vi "HEWH Get UEF.vi"(6 "Maufacturing Date":T1(ring), 7 "Water Heater Type":T7, 8 "error in (no error)":errorcluster, 10 "UEF Calculated Values":T2 {"Data Indexes"."15 sec after Draw Index" format="%#.2f"; "Data Indexes"."15 sec after Draw Timestamp" format="%#.2f"; "Data Indexes"."Test Start Timestamp" format="%.2f"; "Data Indexes"."Test End Timestamp" format="%.2f"; "Data Indexes"."T0 Timestamp" format="%.2f"; "Data Indexes"."Tsf Timestamp" format="%.2f"; "Data Indexes"."Tsu0 Timestamp" format="%.2f"; "Data Indexes"."Tmax1 Timestamp" format="%.2f"; "Data Indexes"."Draw Index Timestamp" format="%#.2f"; "Data Indexes"."Non-Draw Timestamp" format="%#.2f"; "Data Indexes"."Heating Timestamp" format="%#.2f"; "Data Indexes"."Start Energy (BTU-Gas)" format="%.6f"; "Data Indexes"."Start Watt Hours" format="%.6f"; "Static Data"."V - Volume of Wh (True)" format="%.5f"; "Static Data"."T-Ambinet Nominal (°F)" format="%.5f"; "Static Data"."T-Inlet Setpoint (°F)" format="%.5f"; "Static Data"."T-Wh Setpoint (°F)" format="%.5f"; "Sampled Data"."Qe (Wh)" format="%.5f"; "Sampled Data"."Tau stby2 (hr)" format="%.5f"; "Sampled Data"."Tastby2 (°F)" format="%.5f"; "Sampled Data"."Qf (BTU)" format="%.5f"; "Sampled Data"."Qe (BTU)" format="%.5f"; "Sampled Data"."Tmax1 (°F)" format="%.5f"; "Sampled Data"."T0 (°F)" format="%.5f"; "Sampled Data"."Qr (BTU)" format="%.5f"; "Sampled Data"."T 24(°F)" format="%.5f"; "Sampled Data"."T astby(°F)" format="%.5f"; "Sampled Data"."T tstby(°F)" format="%.5f"; "Sampled Data"."T su0(°F)" format="%.5f"; "Sampled Data"."T suf(°F)" format="%.5f"; "Sampled Data"."Tau stby_1 (hr)" format="%.5f"; "Sampled Data"."Qsuf (BTU)" format="%.5f"; "Sampled Data"."Qsu0 (BTU)" format="%.5f"; "Calculated Values"."Draw Bonus Volume (gal)" format="%.6f"; "Calculated Values"."Adjustment Factor" format="%.6f"; "Calculated Values"."T*avg_del(n-1)" format="%.6f"; "Calculated Values"."T*min(n-1)" format="%.6f"; "Calculated Values"."T*avg_del(n)" format="%.6f"; "Calculated Values"."Vn" format="%.6f"; "Calculated Values"."Qdm (BTU)" format="%.6f"; "Calculated Values"."QHWD (BTU)" format="%.6f"; "Calculated Values"."QHW (BTU)" format="%.6f"; "Calculated Values"."UEF" format="%.6f"; "Calculated Values"."QHW67 (BTU)" format="%.6f"; "Calculated Values"."Qda (BTU)" format="%.6f"; "Calculated Values"."Qd (BTU)" format="%.6f"; "Calculated Values"."Q (BTU)" format="%.6f"; "Calculated Values"."UA (BTU/(hr*F))" format="%.6f"; "Calculated Values"."Qhr (BTU/hr)" format="%.6f"; "Calculated Values"."Qstby (BTU)" format="%.6f"; "Calculated Values"."nu_r" format="%.6f"; "Calculated Values"."CpUEF (BTU/(lb*F))" format="%.6f"; "Calculated Values"."rho_nu (lb/gal)" format="%.6f"; "Calculated Values"."V1- Vol (Gal)" format="%.6f"; "Calculated Values"."M cluster mass removed (lb)" format="%.6f"; "Calculated Values"."Cp theoretical (BTU/(lbm °F))" format="%.6f"; "Calculated Values"."Tin1 - Mean Inlet 1st Cluster (°F)" format="%.6f"; "Calculated Values"."Tdel1-Mean Outlet 1st Cluster(°F)" format="%.6f"; "Calculated Values"."Cp 24 (BTU/(lb*F))" format="%.6f"; "Calculated Values"."Cp standby (BTU/(lb*F))" format="%.6f"; "Calculated Values"."Cp2 (BTU/(lb*F))" format="%.6f"; "Calculated Values"."Cp1 (BTU/(lb*F))" format="%.6f"; "Calculated Values"."rho 24 (lb/gal)" format="%.6f"; "Calculated Values"."rho standby (lb/gal)" format="%.6f"; "Calculated Values"."rho 2 (lb/gal)" format="%.6f"; "Calculated Values"."Density of cold water All (lbm/gal)" format="%#.3g"; "Calculated Values"."CpHW (BTU/(lbm °F))" format="%#.3g"; "Calculated Values"."Density of hot water All (lbm/gal)" format="%#.3g"; "Calculated Values"."Mass of water All (lbm)" format="%#.3f"}, 11 "24 Hour UEF Location":path) -> (0 "error out":errorcluster, 2 "UEF Calculated Values Output":T2 {"Data Indexes"."15 sec after Draw Index" format="%#.2f"; "Data Indexes"."15 sec after Draw Timestamp" format="%#.2f"; "Data Indexes"."Test Start Timestamp" format="%.2f"; "Data Indexes"."Test End Timestamp" format="%.2f"; "Data Indexes"."T0 Timestamp" format="%.2f"; "Data Indexes"."Tsf Timestamp" format="%.2f"; "Data Indexes"."Tsu0 Timestamp" format="%.2f"; "Data Indexes"."Tmax1 Timestamp" format="%.2f"; "Data Indexes"."Draw Index Timestamp" format="%#.2f"; "Data Indexes"."Non-Draw Timestamp" format="%#.2f"; "Data Indexes"."Heating Timestamp" format="%#.2f"; "Data Indexes"."Start Energy (BTU-Gas)" format="%.6f"; "Data Indexes"."Start Watt Hours" format="%.6f"; "Static Data"."V - Volume of Wh (True)" format="%.5f"; "Static Data"."T-Ambinet Nominal (°F)" format="%.5f"; "Static Data"."T-Inlet Setpoint (°F)" format="%.5f"; "Static Data"."T-Wh Setpoint (°F)" format="%.5f"; "Sampled Data"."Qe (Wh)" format="%.5f"; "Sampled Data"."Tau stby2 (hr)" format="%.5f"; "Sampled Data"."Tastby2 (°F)" format="%.5f"; "Sampled Data"."Qf (BTU)" format="%.5f"; "Sampled Data"."Qe (BTU)" format="%.5f"; "Sampled Data"."Tmax1 (°F)" format="%.5f"; "Sampled Data"."T0 (°F)" format="%.5f"; "Sampled Data"."Qr (BTU)" format="%.5f"; "Sampled Data"."T 24(°F)" format="%.5f"; "Sampled Data"."T astby(°F)" format="%.5f"; "Sampled Data"."T tstby(°F)" format="%.5f"; "Sampled Data"."T su0(°F)" format="%.5f"; "Sampled Data"."T suf(°F)" format="%.5f"; "Sampled Data"."Tau stby_1 (hr)" format="%.5f"; "Sampled Data"."Qsuf (BTU)" format="%.5f"; "Sampled Data"."Qsu0 (BTU)" format="%.5f"; "Calculated Values"."Draw Bonus Volume (gal)" format="%.6f"; "Calculated Values"."Adjustment Factor" format="%.6f"; "Calculated Values"."T*avg_del(n-1)" format="%.6f"; "Calculated Values"."T*min(n-1)" format="%.6f"; "Calculated Values"."T*avg_del(n)" format="%.6f"; "Calculated Values"."Vn" format="%.6f"; "Calculated Values"."Qdm (BTU)" format="%.6f"; "Calculated Values"."QHWD (BTU)" format="%.6f"; "Calculated Values"."QHW (BTU)" format="%.6f"; "Calculated Values"."UEF" format="%.6f"; "Calculated Values"."QHW67 (BTU)" format="%.6f"; "Calculated Values"."Qda (BTU)" format="%.6f"; "Calculated Values"."Qd (BTU)" format="%.6f"; "Calculated Values"."Q (BTU)" format="%.6f"; "Calculated Values"."UA (BTU/(hr*F))" format="%.6f"; "Calculated Values"."Qhr (BTU/hr)" format="%.6f"; "Calculated Values"."Qstby (BTU)" format="%.6f"; "Calculated Values"."nu_r" format="%.6f"; "Calculated Values"."CpUEF (BTU/(lb*F))" format="%.6f"; "Calculated Values"."rho_nu (lb/gal)" format="%.6f"; "Calculated Values"."V1- Vol (Gal)" format="%.6f"; "Calculated Values"."M cluster mass removed (lb)" format="%.6f"; "Calculated Values"."Cp theoretical (BTU/(lbm °F))" format="%.6f"; "Calculated Values"."Tin1 - Mean Inlet 1st Cluster (°F)" format="%.6f"; "Calculated Values"."Tdel1-Mean Outlet 1st Cluster(°F)" format="%.6f"; "Calculated Values"."Cp 24 (BTU/(lb*F))" format="%.6f"; "Calculated Values"."Cp standby (BTU/(lb*F))" format="%.6f"; "Calculated Values"."Cp2 (BTU/(lb*F))" format="%.6f"; "Calculated Values"."Cp1 (BTU/(lb*F))" format="%.6f"; "Calculated Values"."rho 24 (lb/gal)" format="%.6f"; "Calculated Values"."rho standby (lb/gal)" format="%.6f"; "Calculated Values"."rho 2 (lb/gal)" format="%.6f"; "Calculated Values"."Density of cold water All (lbm/gal)" format="%#.3g"; "Calculated Values"."CpHW (BTU/(lbm °F))" format="%#.3g"; "Calculated Values"."Density of hot water All (lbm/gal)" format="%#.3g"; "Calculated Values"."Mass of water All (lbm)" format="%#.3f"}, 3 "24 Hour UEF Location Output":path, 4 "Full 24 Hour UEF Data":string[][](array[string]))   [LabVIEW 2023]
uses:
  Type Definitions/HEWH Water Heater Type.ctl
  Type Definitions/UEF Constants.ctl
  Type Definitions/HEWH Draw Stats.ctl
  Type Definitions/HEWH FHR Draw Type.ctl
  Type Definitions/FHR Bins.ctl
  Type Definitions/HEWH Meter Type.ctl
  Type Definitions/HEWH Test Type.ctl
  Type Definitions/HEWH Index Type.ctl
  <vilib>/Utility/file.llb/Read Delimited Spreadsheet (string).vi
  <vilib>/Utility/file.llb/Read Delimited Spreadsheet (DBL).vi
panel:
  # "FHR"
  # "FHR"
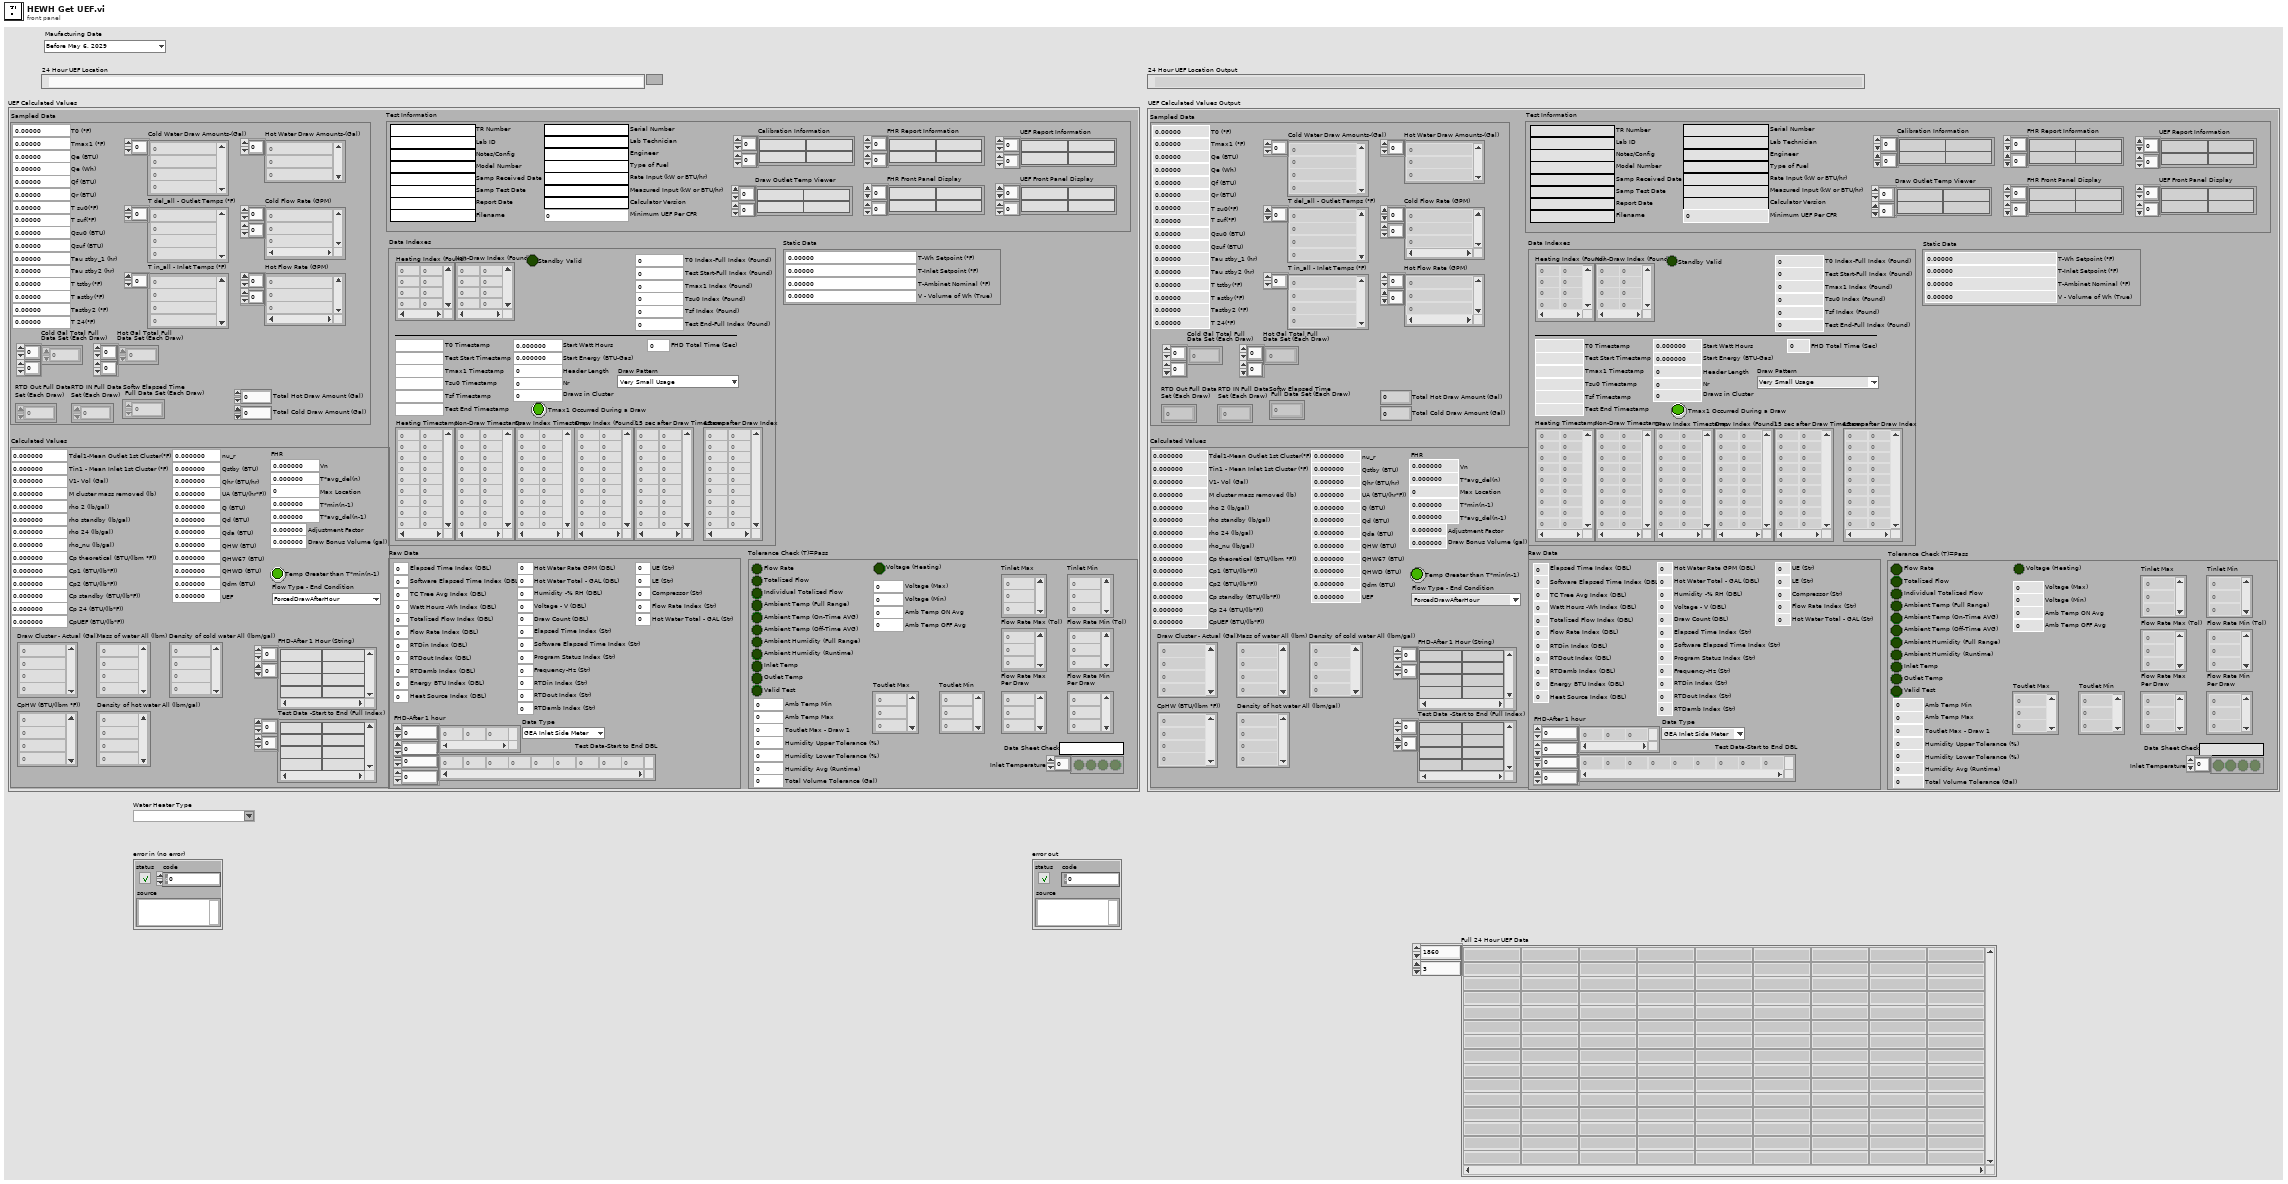
[diagram p1: front panel]
types:
  T1 = enum16{"Before May 6, 2029", "On or After May 6, 2029"}
  T2 = typedef "UEF Constants.ctl" = cluster{"Calculated Values":T3, "Sampled Data":cluster{"Cold Water Draw Amounts-(Gal)":dbl[], "T del_all - Outlet Temps (°F)":dbl[], "T in_all - Inlet Temps (°F)":dbl[], "Qsu0 (BTU)":dbl, "Qsuf (BTU)":dbl, "Tau stby_1 (hr)":dbl, "T suf(°F)":dbl, "T su0(°F)":dbl, "T tstby(°F)":dbl, "T astby(°F)":dbl, "T 24(°F)":dbl, "Qr (BTU)":dbl, "T0 (°F)":dbl, "Tmax1 (°F)":dbl, "Qe (BTU)":dbl, "Qf (BTU)":dbl, "Tastby2 (°F)":dbl, "RTD Out Full Data\nSet (Each Draw)":dbl[][], "RTD IN Full Data\nSet (Each Draw)":dbl[][], "Tau stby2 (hr)":dbl, "Hot Water Draw Amounts-(Gal)":dbl[], "Cold Flow Rate (GPM)":dbl[][], "Hot Flow Rate (GPM)":dbl[][], "Softw Elapsed Time\n Full Data Set (Each Draw)":dbl[][], "Cold Gal Total Full\nData Set (Each Draw)":dbl[][], "Total Hot Draw Amount (Gal) ":dbl, "Total Cold Draw Amount (Gal)":dbl, "Qe (Wh)":dbl, "Hot Gal Total Full\nData Set (Each Draw)":dbl[][]}, "Static Data":cluster{"T-Wh Setpoint (°F)":dbl, "T-Inlet Setpoint (°F)":dbl, "T-Ambinet Nominal (°F)":dbl, "V - Volume of Wh (True)":dbl}, "Data Indexes":cluster{"Test Start-Full Index (Found)":i32, "Header Length":i32, "Draw Index (Found)":i32[][], "Nr":i32, "Start Watt Hours":dbl, "Tsu0 Index (Found)":i32, "Tsf Index (Found)":i32, "Start Energy (BTU-Gas)":dbl, "Draws in Cluster":i32, "T0 Index-Full Index (Found)":i32, "Non-Draw Index (Found)":i32[][], "Tmax1 Index (Found)":i32, "Test End-Full Index (Found)":i32, "Heating Index (Found)":i32[][], "Heating Timestamp":dbl[][], "Non-Draw Timestamp":dbl[][], "Draw Index Timestamp":dbl[][], "Tmax1 Timestamp":dbl, "Tsu0 Timestamp":dbl, "Tsf Timestamp":dbl, "T0 Timestamp":dbl, "Test End Timestamp":dbl, "Test Start Timestamp":dbl, "15 sec after Draw Timestamp":dbl[][], "15 sec after Draw Index":dbl[][], "Tmax1 Occurred During a Draw":bool, "FHD Total Time (Sec)":dbl, "Draw Pattern":T5, "Standby Valid":bool}, "Raw Data":cluster{"Elapsed Time Index (DBL)":i32, "Software Elapsed Time Index (DBL)":i32, "TC Tree Avg Index (DBL)":i32, "Watt Hours -Wh Index (DBL)":i32, "Energy BTU Index (DBL)":i32, "Totalized Flow Index (DBL)":i32, "Flow Rate Index (DBL)":i32, "Program Status Index (Str)":i32, "RTDin Index (DBL)":i32, "RTDout Index (DBL)":i32, "RTDamb Index (DBL)":i32, "Test Data-Start to End DBL":dbl[][], "Data Type":T6, "Heat Source Index (DBL)":i32, "Hot Water Rate GPM (DBL)":i32, "Hot Water Total - GAL (DBL)":i32, "FHD-After 1 hour":dbl[][], "Humidity -% RH (DBL)":i32, "Voltage - V (DBL)":i32, "Draw Count (DBL)":i32, "Elapsed Time Index (Str)":i32, "Software Elapsed Time Index (Str)":i32, "Frequency-Hz (Str)":i32, "RTDin Index (Str)":i32, "RTDout Index (Str)":i32, "RTDamb Index (Str)":i32, "UE (Str)":i32, "LE (Str)":i32, "Compressor (Str)":i32, "Flow Rate Index (Str)":i32, "Hot Water Total - GAL (Str)":i32}, "Tolerance Check (T)=Pass":cluster{"Flow Rate":bool, "Totalized Flow":bool, "Ambient Temp (Full Range)":bool, "Ambient Humidity (Full Range)":bool, "Inlet Temp":bool, "Outlet Temp":bool, "Valid Test":bool, "Individual Totalized Flow":bool, "Data Sheet Check":string, "Inlet Temperature":bool[], "Tinlet Max":dbl[], "Tinlet Min":dbl[], "Flow Rate Max (Tol)":dbl[], "Flow Rate Min (Tol)":dbl[], "Amb Temp Max":dbl, "Amb Temp Min":dbl, "Toutlet Max - Draw 1":dbl, "Humidity Upper Tolerance (%)":dbl, "Total Volume Tolerance (Gal)":dbl, "Humidity Lower Tolerance (%)":dbl, "Flow Rate Max\nPer Draw":dbl[], "Flow Rate Min\nPer Draw":dbl[], "Ambient Humidity (Runtime)":bool, "Humidity Avg (Runtime)":dbl, "Ambient Temp (On-Time AVG)":bool, "Ambient Temp (Off-Time AVG)":bool, "Amb Temp OFF Avg":dbl, "Amb Temp ON Avg":dbl, "Voltage (Heating)":bool, "Voltage (Min)":dbl, "Voltage (Max)":dbl, "Toutlet Max":dbl[], "Toutlet Min":dbl[]}, "Test Information":cluster{"TR Number":string, "Lab ID":string, "Notes/Config":string, "Model Number":string, "Serial Number":string, "Lab Technician":string, "Engineer":string, "Type of Fuel":string, "Samp Received Date":string, "Samp Test Date":string, "Report Date":string, "Rate Input (kW or BTU/hr)":string, "Measured Input (kW or BTU/hr)":string, "Filename":string, "Calibration Information":string[][], "Calculator Version":string, "Minimum UEF Per CFR":dbl, "UEF Report Information":string[][], "FHR Report Information":string[][], "FHR Front Panel Display":string[][], "UEF Front Panel Display":string[][], "Draw Outlet Temp Viewer":string[][]}}
  T3 = typedef "HEWH Draw Stats.ctl" = cluster{"Draw Cluster - Actual (Gal)":dbl[], "Mass of water All (lbm)":dbl[], "Density of hot water All (lbm/gal)":dbl[], "CpHW (BTU/(lbm °F))":dbl[], "rho 2 (lb/gal)":dbl, "rho standby (lb/gal)":dbl, "rho 24 (lb/gal)":dbl, "Cp1 (BTU/(lb*F))":dbl, "Cp2 (BTU/(lb*F))":dbl, "Cp standby (BTU/(lb*F))":dbl, "Cp 24 (BTU/(lb*F))":dbl, "nu_r":dbl, "Qstby (BTU)":dbl, "Qhr (BTU/hr)":dbl, "UA (BTU/(hr*F))":dbl, "Q (BTU)":dbl, "Qd (BTU)":dbl, "Qda (BTU)":dbl, "QHW67 (BTU)":dbl, "UEF":dbl, "Tdel1-Mean Outlet 1st Cluster(°F)":dbl, "Tin1 - Mean Inlet 1st Cluster (°F)":dbl, "Cp theoretical (BTU/(lbm °F))":dbl, "M cluster mass removed (lb)":dbl, "V1- Vol (Gal)":dbl, "Test Data -Start to End (Full Index)":string[][], "rho_nu (lb/gal)":dbl, "Density of cold water All (lbm/gal)":dbl[], "CpUEF (BTU/(lb*F))":dbl, "QHW (BTU)":dbl, "QHWD (BTU)":dbl, "Qdm (BTU)":dbl, "FHD-After 1 Hour (String)":string[][], "Vn":dbl, "T*avg_del(n)":dbl, "Max Location":i32, "T*min(n-1)":dbl, "T*avg_del(n-1)":dbl, "Temp Greater than T*min(n-1)":bool, "Adjustment Factor":dbl, "Draw Bonus Volume (gal)":dbl, "Flow Type - End Condition":T4}
  T4 = typedef "HEWH FHR Draw Type.ctl" = enum16{"ForcedDrawAfterHour", "HeatingCutoffBeforeHour"}
  T5 = typedef "FHR Bins.ctl" = enum16{"Very Small Usage", "Low Usage", "Medium Usage", "High Usage", "Undefined"}
  T6 = typedef "HEWH Meter Type.ctl" = enum16{"GEA Inlet Side Meter", "GEA Outlet Side Meter", "CSA Inlet Side Meter"}
  T7 = typedef "HEWH Water Heater Type.ctl" = string
  T8 = typedef "HEWH Index Type.ctl" = enum16{"Draw Index", "Heating Index", "Temp Based (FHD)"}
  T9 = typedef "HEWH Test Type.ctl" = enum16{"UEF", "FHD"}
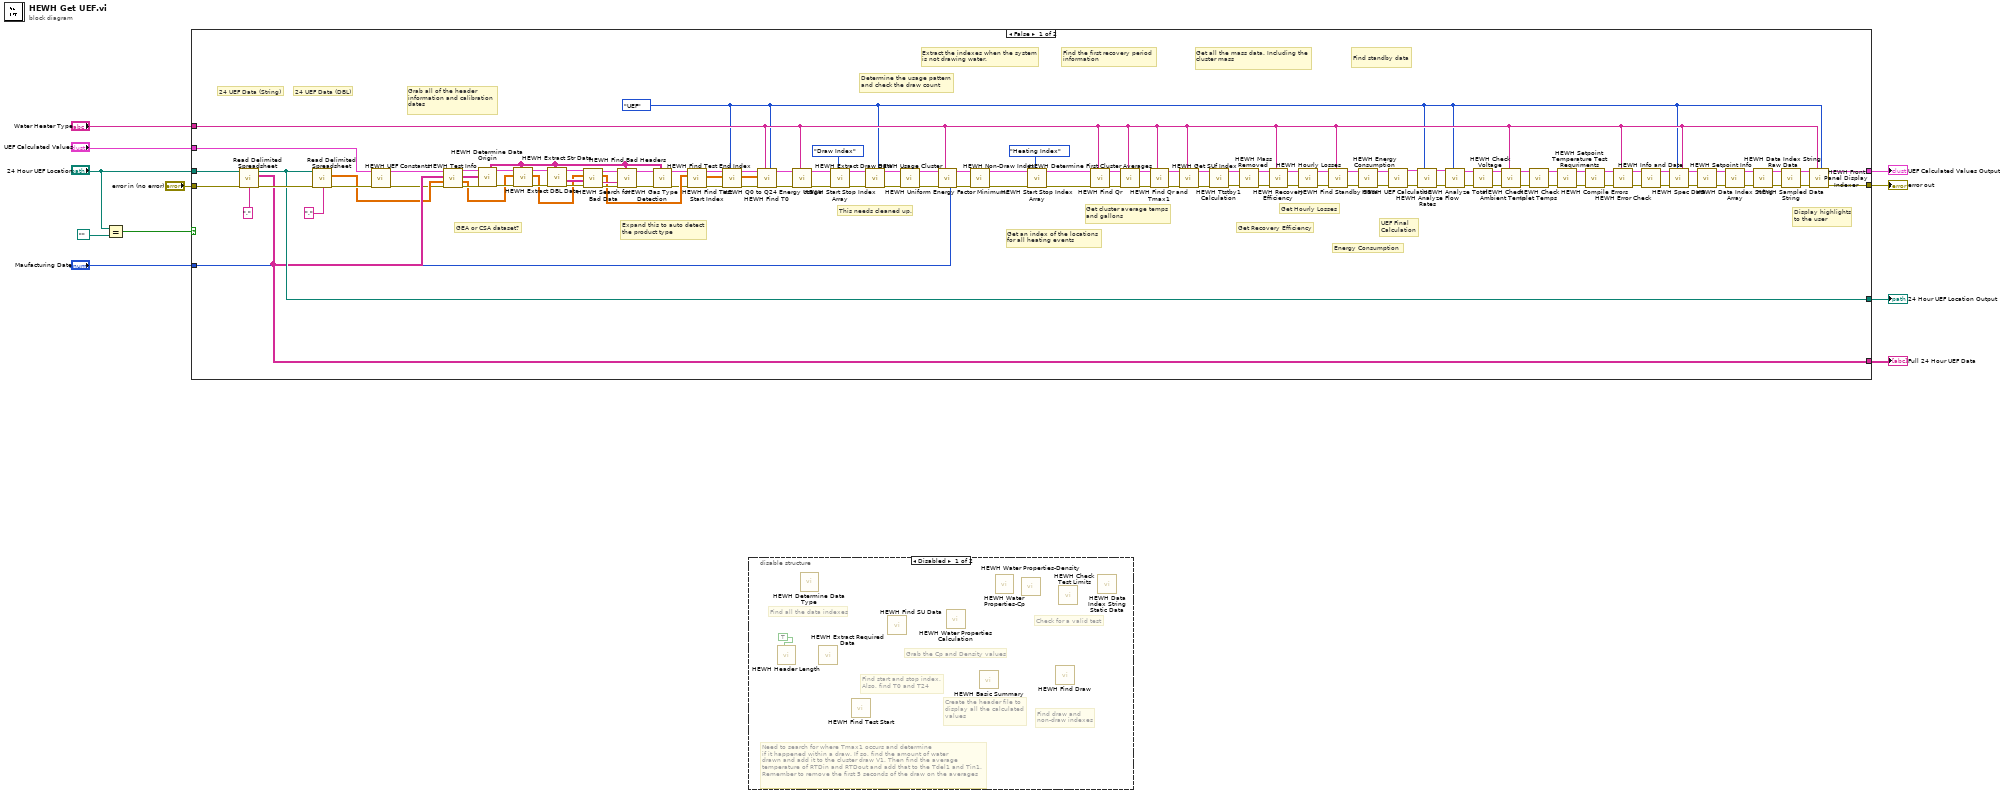
[diagram p0: block diagram]
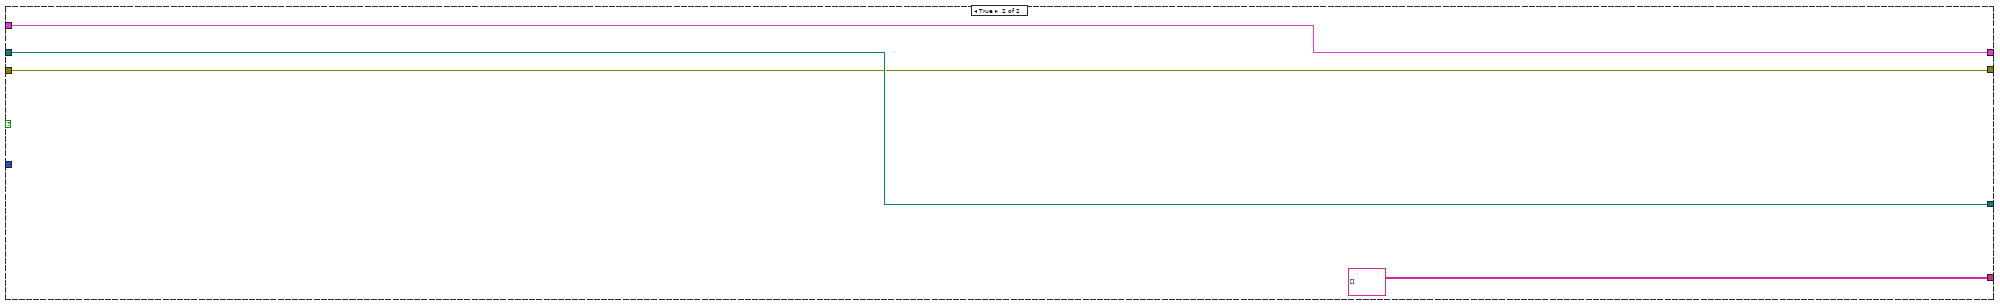
[diagram p3: hidden frame]
diagram:
  n1 = Equal?(x="24 Hour UEF Location", y=path "") -> (x = y?=w2:bool)
  n2 = case shown="False" w2 {
    tunnel: "Water Heater Type" -> [w15 _]
    tunnel: "UEF Calculated Values" -> [w88 w125]
    tunnel: [w54 string[][] [] ("all rows")] -> w9
    tunnel: "error in (no error)" -> [w123 w126]
    tunnel: [w107 w126] -> w7
    tunnel: [w12 w125] -> w6
    tunnel: [w108 w127] -> w5
    tunnel: "24 Hour UEF Location" -> [w109 w127]
    tunnel: "Maufacturing Date" -> [w46 _]
    frame False {
      w13 = HEWH_Test_Type."UEF" ("Test Type")
      # "Expand this to auto detect\nthe product type"
      # "This needs cleaned up."
      # "Determine the usage pattern\nand check the draw count"
      # "Get an index of the locations \nfor all heating events"
      # "Extract the indexes when the system\nis not drawing water."
      # "GEA or CSA dataset?"
      # "Grab all of the header\ninformation and calibration\ndates"
      # "Display highlights\nto the user"
      # "UEF Final\nCalculation"
      # "Energy Consumption"
      # "Find standby data"
      # "Get Hourly Losses"
      # "Get Recovery Efficiency"
      # "24 UEF Data (DBL)"
      # "24 UEF Data (String)"
      # "Get cluster average temps\nand gallons"
      # "Get all the mass data. Including the \ncluster mass"
      # "Find the first recovery period\ninformation"
      n3 = call-poly <vilib>:"Read Delimited Spreadsheet.vi"("file path (dialog if empty)"=w109, "error in (no error)"=w123, "delimiter (\\t)"="," ("delimiter (\\t)")) -> ("new file path (Not A Path if cancelled)"=w108:path, "all rows"=w54:string[][], "error out"=w122:errorcluster)  [unwired: 7 in, 3 out]
      n4 = call-poly <vilib>:"Read Delimited Spreadsheet.vi"("file path (dialog if empty)"=w108, "error in (no error)"=w122, "delimiter (\\t)"="," ("delimiter (\\t)")) -> ("all rows"=w53:dbl[][], "error out"=w87:errorcluster)  [unwired: 7 in, 4 out]
      n5 = call "HEWH UEF Constants.vi"("error in (no error)"=w87, "UEF Calculated Values Input"=w88) -> ("error out"=w51:errorcluster, "UEF Calculated Values Output"=w55:T2)  [unwired: 8 in]
      n6 = call "HEWH Test Info.vi"("error in (no error)"=w51, "Full Data DBL"=w53, "Full Data (String)"=w54, "UEF Calculated Values Input"=w55) -> ("error out"=w85:errorcluster, "Full Data DBL Out"=w52:dbl[][], "Full Data (String)"=w86:string[][], "UEF Calculated Values Output"=w50:T2)  [unwired: 4 in]
      n7 = call "HEWH Determine Data Origin.vi"("error in (no error)"=w85, "Full Data (String)"=w86, "UEF Calculated Values Output in"=w50) -> ("error out"=w59:errorcluster, "UEF Calculated Values Output out"=w56:T2, "Full Data (String) Out"=w62:string[][])  [unwired: 6 in]
      n8 = call "HEWH Extract DBL Data.vi"("Full Data (String)"=w62, "error in (no error)"=w59, "Full Data DBL In"=w52, "UEF Calculated Values Input in"=w56) -> ("error out"=w69:errorcluster, "Full Data DBL Out"=w61:dbl[][], "UEF Calculated Values Input out"=w66:T2)  [unwired: 5 in]
      n9 = call "HEWH Extract Str Data.vi"("Full Data (String)"=w62, "error in (no error)"=w69, "UEF Calculated Values Input in"=w66) -> ("error out"=w68:errorcluster, "Full Data (String) Out"=w67:string[][], "UEF Calculated Values Input out"=w65:T2)  [unwired: 6 in]
      n10 = call "HEWH Search for Bad Data.vi"("UEF Calculated Values Input"=w65, "Full DBL Array"=w61, "Full String Array"=w67, "error in (no error)"=w68) -> ("UEF Calculated Values Output"=w72:T2, "Full DBL Array Out"=w60:dbl[][], "Message String 1"=w64:string, "error out"=w71:errorcluster)  [unwired: 8 in]
      n11 = call "HEWH Find Bad Headers.vi"("Full Data (String)"=w62, "error in (no error)"=w71, "Message String 1"=w64, "UEF Calculated Values Input"=w72) -> ("error out"=w70:errorcluster, "UEF Calculated Values Output"=w63:T2)  [unwired: 6 in]
      n12 = call "HEWH Gas Type Detection.vi"("Full Data (String)"=w62, "error in (no error)"=w70, "UEF Calculated Values Input"=w63) -> ("error out"=w58:errorcluster, "UEF Calculated Values Output"=w57:T2)  [unwired: 7 in]
      n13 = call "HEWH Find Test Start Index.vi"("error in (no error)"=w58, "Full Data DBL"=w60, "UEF Calculated Values"=w57) -> ("error out"=w89:errorcluster, "Full Data DBL Out"=w92:dbl[][], "UEF Calculated Values Output"=w90:T2)  [unwired: 6 in]
      n14 = call "HEWH Find Test End Index.vi"("Test Type"=w13, "error in (no error)"=w89, "Full Data DBL"=w92, "UEF Calculated Values in"=w90) -> ("error out"=w91:errorcluster, "Full Data DBL Out"=w94:dbl[][], "UEF Calculated Values out"=w93:T2)  [unwired: 5 in]
      n15 = call "HEWH Find T0.vi"("Test Type"=w13, "Water Heater Type"=w15, "Error In"=w91, "Full Data DBL"=w94, "UEF Calculated Values"=w93) -> ("Error Out"=w96:errorcluster, "UEF Calculated Values (Output)"=w95:T2)  [unwired: 4 in, 1 out]
      n16 = call "HEWH Q0 to Q24 Energy Usage.vi"("Water Heater Type"=w15, "error in (no error)"=w96, "UEF Calculated Values (Output) in"=w95) -> ("error out"=w75:errorcluster, "UEF Calculated Values (Output) out"=w76:T2)  [unwired: 7 in]
      n17 = call "HEWH Start Stop Index Array.vi"("Index Type"=HEWH_Index_Type."Draw Index", "error in (no error)"=w75, "UEF Calculated Values in"=w76) -> ("error out"=w81:errorcluster, "UEF Calculated Values Output"=w82:T2)  [unwired: 7 in]
      n18 = call "HEWH Extract Draw Data.vi"("Test Type"=w13, "error in (no error)"=w81, "UEF Calculated Values in"=w82) -> ("error out"=w84:errorcluster, "UEF Calculated Values Out"=w83:T2)  [unwired: 7 in]
      n19 = call "HEWH Usage Cluster.vi"("error in (no error)"=w84, "UEF Calculated Values Output"=w83) -> ("error out"=w49:errorcluster, "UEF Calculated Values out"=w47:T2)  [unwired: 8 in]
      n20 = call "HEWH Uniform Energy Factor Minimums.vi"("Maufacturing Date"=w46, "Water Heater Type"=w15, "error in (no error)"=w49, "UEF Calculated Values Input"=w47) -> ("error out"=w48:errorcluster, "UEF Calculated Values Output"=w45:T2)  [unwired: 6 in]
      n21 = call "HEWH Non-Draw Index.vi"("error in (no error)"=w48, "UEF Calculated Values"=w45) -> ("error out"=w78:errorcluster, "UEF Calculated Values Output"=w77:T2)  [unwired: 8 in]
      n22 = call "HEWH Start Stop Index Array.vi"("Index Type"=HEWH_Index_Type."Heating Index", "error in (no error)"=w78, "UEF Calculated Values in"=w77) -> ("error out"=w73:errorcluster, "UEF Calculated Values Output"=w74:T2)  [unwired: 7 in]
      n23 = call "HEWH Find Qr.vi"("Water Heater Type"=w15, "Error In"=w73, "UEF Calculated Values"=w74) -> ("Error Out"=w102:errorcluster, "UEF Calculated Values Output"=w99:T2)  [unwired: 7 in]
      n24 = call "HEWH Determine First Cluster Averages.vi"("Water Heater Type"=w15, "error in (no error)"=w102, "UEF Calculated Values Input"=w99) -> ("error out"=w101:errorcluster, "UEF Calculated Values Output"=w100:T2)  [unwired: 7 in]
      n25 = call "HEWH Find Qr and Tmax1.vi"("Water Heater Type"=w15, "error in (no error)"=w101, "UEF Calculated Values"=w100) -> ("error out"=w105:errorcluster, "UEF Calculated Values Output"=w106:T2)  [unwired: 7 in]
      n26 = call "HEWH Get SUf Index.vi"("Water Heater Type"=w15, "error in (no error)"=w105, "UEF Calculated Values"=w106) -> ("error out"=w103:errorcluster, "UEF Calculated Values Output"=w104:T2)  [unwired: 7 in]
      n27 = call "HEWH Ttstby1 Calculation.vi"("error in (no error)"=w103, "UEF Calculated Values Output in"=w104) -> ("error out"=w98:errorcluster, "UEF Calculated Values Output out"=w97:T2)  [unwired: 8 in]
      n28 = call "HEWH Mass Removed.vi"("Error In"=w98, "UEF Calculated Values Output in"=w97) -> ("Error Out"=w111:errorcluster, "UEF Calculated Values Output out"=w112:T2)  [unwired: 8 in]
      n29 = call "HEWH Recovery Efficiency.vi"("Water Heater Type"=w15, "Error In"=w111, "UEF Calculated Values Output in"=w112) -> ("Error Out"=w113:errorcluster, "UEF Calculated Values Output"=w114:T2)  [unwired: 7 in]
      n30 = call "HEWH Hourly Losses.vi"("Error In"=w113, "UEF Calculated Values Output in"=w114) -> ("Error Out"=w116:errorcluster, "UEF Calculated Values Output out"=w115:T2)  [unwired: 8 in]
      n31 = call "HEWH Find Standby Data.vi"("Water Heater Type"=w15, "error in (no error)"=w116, "UEF Calculated Values Input"=w115) -> ("error out"=w118:errorcluster, "UEF Calculated Values Output"=w117:T2)  [unwired: 7 in]
      n32 = call "HEWH Energy Consumption.vi"("Error In"=w118, "UEF Calculated Values Output in"=w117) -> ("Error Out"=w119:errorcluster, "UEF Calculated Values Output"=w120:T2)  [unwired: 8 in]
      n33 = call "HEWH UEF Calculation.vi"("Error In"=w119, "UEF Calculated Values"=w120) -> ("Error Out"=w34:errorcluster, "UEF Calculated Values Output"=w33:T2)  [unwired: 8 in]
      n34 = call "HEWH Analyze Flow Rates.vi"("UEF Calculated Values Input"=w33, "Test Type"=w13, "error in (no error)"=w34) -> ("UEF Calculated Values Output"=w42:T2, "error out"=w41:errorcluster)  [unwired: 11 in]
      n35 = call "HEWH Analyze Total.vi"("Test Type"=w13, "error in (no error)"=w41, "UEF Calculated Values Input"=w42) -> ("error out"=w43:errorcluster, "UEF Calculated Values Output"=w44:T2)  [unwired: 7 in]
      n36 = call "HEWH Check Voltage.vi"("error in (no error)"=w43, "UEF Calculated Values Input"=w44) -> ("error out"=w35:errorcluster, "UEF Calculated Values Output"=w36:T2)  [unwired: 8 in]
      n37 = call "HEWH Check Ambient Temp.vi"("Water Heater Type"=w15, "error in (no error)"=w35, "UEF Calculated Values Input"=w36) -> ("error out"=w37:errorcluster, "UEF Calculated Values Output"=w39:T2)  [unwired: 7 in]
      n38 = call "HEWH Check Inlet Temps.vi"("error in (no error)"=w37, "UEF Calculated Values Input"=w39) -> ("error out"=w38:errorcluster, "UEF Calculated Values Output"=w40:T2)  [unwired: 8 in]
      n39 = call "HEWH Setpoint Temperature Test Requriments.vi"("error in"=w38, "UEF Calculated Values Input"=w40) -> ("error out"=w31:errorcluster, "UEF Calculated Values Output"=w32:T2)  [unwired: 8 in]
      n40 = call "HEWH Compile Errors.vi"("error in (no error)"=w31, "UEF Calculated Values Input"=w32) -> ("error out"=w29:errorcluster, "UEF Calculated Values Output"=w30:T2)  [unwired: 8 in]
      n41 = call "HEWH Error Check.vi"("Water Heater Type"=w15, "error in (no error)"=w29, "UEF Calculated Values Output in"=w30) -> ("error out"=w19:errorcluster, "UEF Calculated Values Output"=w17:T2)  [unwired: 7 in]
      n42 = call "HEWH Info and Date.vi"("error in (no error)"=w19, "UEF Calculated Values Output in"=w17) -> ("error out"=w21:errorcluster, "UEF Calculated Values Output out"=w20:T2)  [unwired: 8 in]
      n43 = call "HEWH Spec Data.vi"("Water Heater Type"=w15, "Test Type"=w13, "error in (no error)"=w21, "UEF Calculated Values Input"=w20) -> ("error out"=w22:errorcluster, "UEF Calculated Values Output"=w23:T2)  [unwired: 6 in]
      n44 = call "HEWH Setpoint Info.vi"("error in (no error)"=w22, "UEF Calculated Values Input"=w23) -> ("error out"=w18:errorcluster, "UEF Calculated Values Output"=w16:T2)  [unwired: 8 in]
      n45 = call "HEWH Data Index String Array.vi"("error in (no error)"=w18, "UEF Calculated Values Input"=w16) -> ("error out"=w25:errorcluster, "UEF Calculated Values Output"=w26:T2)  [unwired: 8 in]
      n46 = call "HEWH Data Index String Raw Data.vi"("error in (no error)"=w25, "UEF Calculated Values Input"=w26) -> ("error out"=w28:errorcluster, "UEF Calculated Values Output"=w27:T2)  [unwired: 8 in]
      n47 = call "HEWH Sampled Data String.vi"("error in (no error)"=w28, "UEF Calculated Values Output in"=w27) -> ("error out"=w24:errorcluster, "UEF Calculated Values Output out"=w14:T2)  [unwired: 8 in]
      n48 = call "HEWH Front Panel Display Indexer.vi"("Test Type"=w13, "Water Heater Type"=w15, "error in (no error)"=w24, "UEF Calculated Values Input"=w14) -> ("error out"=w107:errorcluster, "UEF Calculated Values Output"=w12:T2)  [unwired: 6 in]
    }
    frame True {
    }
  }
  "Full 24 Hour UEF Data" <- w9
  "error out" <- w7
  "UEF Calculated Values Output" <- w6
  "24 Hour UEF Location Output" <- w5
  n49 = disable-structure shown="Disabled" {
    frame Disabled {
      # "Create the header file to \ndisplay all the calculated \nvalues"
      # "Check for a valid test"
      # "Find draw and \nnon-draw indexes"
      # "Find all the data indexes"
      # "Need to search for where Tmax1 occurs and determine \nif it happened within a draw. If so, find the amount of water\ndrawn and add it to the cluster draw V1. Then find the average \ntemperature of RTDin and RTDout and add that to the Tdel1 and Tin1.\nRemember to remove the first 5 seconds of the draw on the averages"
      # "Find start and stop index.\nAlso, find T0 and T24"
      # "Grab the Cp and Density values"
      n50 = call "HEWH Header Length.vi"("DBL?"=TRUE) -> ()  [unwired: 7 in, 4 out]
      n51 = call "HEWH Determine Data Type.vi"() -> ()  [unwired: 9 in, 3 out]
      n52 = call "HEWH Extract Required Data.vi"() -> ()  [unwired: 9 in, 3 out]
      n53 = call "HEWH Find Test Start.vi"() -> ()  [unwired: 10 in, 2 out]
      n54 = call "HEWH Find SU Data.vi"() -> ()  [unwired: 10 in, 2 out]
      n55 = call "HEWH Water Properties Calculation.vi"() -> ()  [unwired: 10 in, 2 out]
      n56 = call "HEWH Basic Summary.vi"() -> ()  [unwired: 9 in, 3 out]
      n57 = call "HEWH Water Properties-Cp.vi"() -> ()  [unwired: 10 in, 2 out]
      n58 = call "HEWH Water Properties-Density.vi"() -> ()  [unwired: 10 in, 2 out]
      n59 = call "HEWH Find Draw.vi"() -> ()  [unwired: 10 in, 2 out]
      n60 = call "HEWH Check Test Limits.vi"() -> ()  [unwired: 9 in, 3 out]
      n61 = call "HEWH Data Index String Static Data.vi"() -> ()  [unwired: 10 in, 2 out]
    }
    frame Enabled {
    }
  }
